vi "pco.camera_Simple_Example_IMAQ.vi"() -> ()   [LabVIEW 2019]
uses:
  pco.camera/Camera.lvclass
panel:
  out "rawImage":u16[][](array[numeric])
  out "Image":T1(plugin-control)
  in  "data_format":T2(ring)=enum."Mono16"
  in  "Image Index":u32 max=99
  out "Recorded Images":u32
  in  "Quit":bool
  in  "roiY1":u64=2 min=2 max=1040 step=1
  in  "roiX1":u64=2 min=2 max=1392 step=1
  in  "roiY0":u64=1 min=1 max=1039 step=1
  in  "roiX0":u64=1 min=1 max=1391 step=1
  out "Image Height":u16
  out "Image Width":u16
  in  "dwImgCount":u32=10 caption="Required Number of Images" max=4023
  out "Error":errorcluster {"code" format="%x"}
  # "This example shows a simple recording of an image sequence and the image access afterwards.\nIt is a good starting point for writing own applications.\nBut it will not be fail save, i.e. doesnt react on errors, just handles them forward to the end\n\nUsage:\nSelect your required image count before you start the program.\nOnce started, the camera class will be initialized and images will be recorded automatically.\nWhen acquisition has finished you can address the images and set a certain roi \nTo finish the program click on quit application, this will force fan exit of the camera class"
  # "pco.labview"
  # "Camera Setup"
  # "Recording Control"
  # "Parameters for image readout"
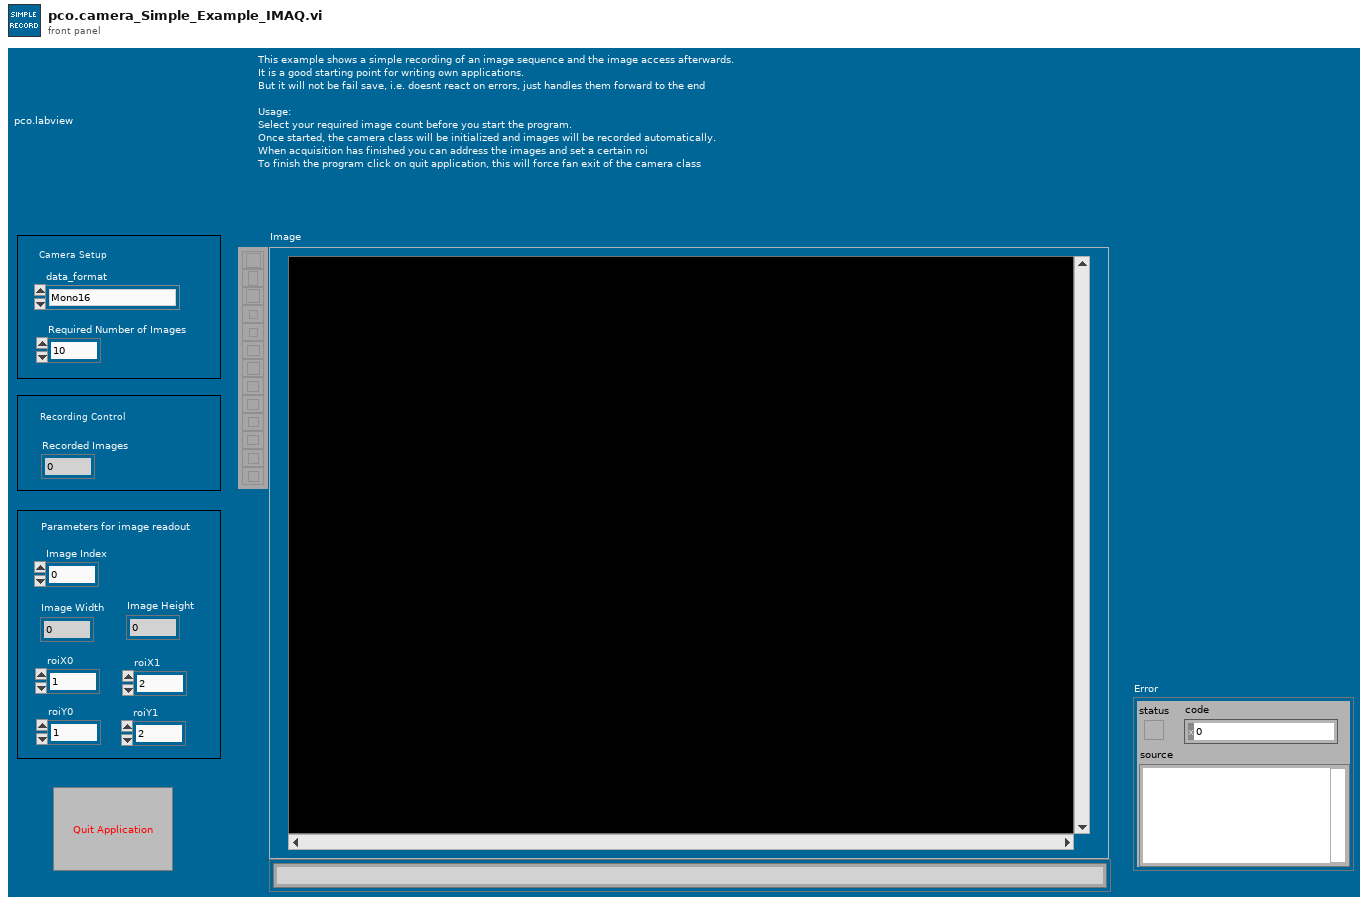
[diagram p1: front panel]
types:
  T1 = typedef "IMAQ Image.ctl" = refnum<image>
  T2 = enum16{"Undefined", "Mono8", "Mono16", "BGRA8", "RGBA8", "BGRA16", "RGBA16", "CompressedMono8"}
  T3 = enum8{"Enabled", "Disabled", "Disabled and Grayed Out"}
  T4 = enum16{"sequence", "sequence non blocking", "ring buffer", "fifo", "sequence_dpcore", "sequence_non_blocking_dpcore", "ring_buffer_dpcore", "fifo_dpcore", "tif", "multitif", "pcoraw", "b16", "dicom", "multidicom"}
  T5 = typedef "Image Type" = u32
  T6 = typedef "Camera.lvclass/binning.ctl" = cluster{"vert":u16, "horz":u16}
  T7 = cluster{"exposure_time_s":dbl, "delay_time_s":dbl, "roi":cluster{"x0":u64, "y0":u64, "x1":u64, "y1":u64}, "timestamp_mode":u16, "pixelrate":u32, "trigger_mode":u16, "acquire_mode":u16, "metadata_mode":u16, "noisefilter_mode":u16, "binning":T6}
  T8 = typedef "Color (U64)" = cluster{"Plane 3 (Blue)":u16, "Plane 2 (Green)":u16, "Plane 1 (Red)":u16, "Plane 4 (alpha)":u16}
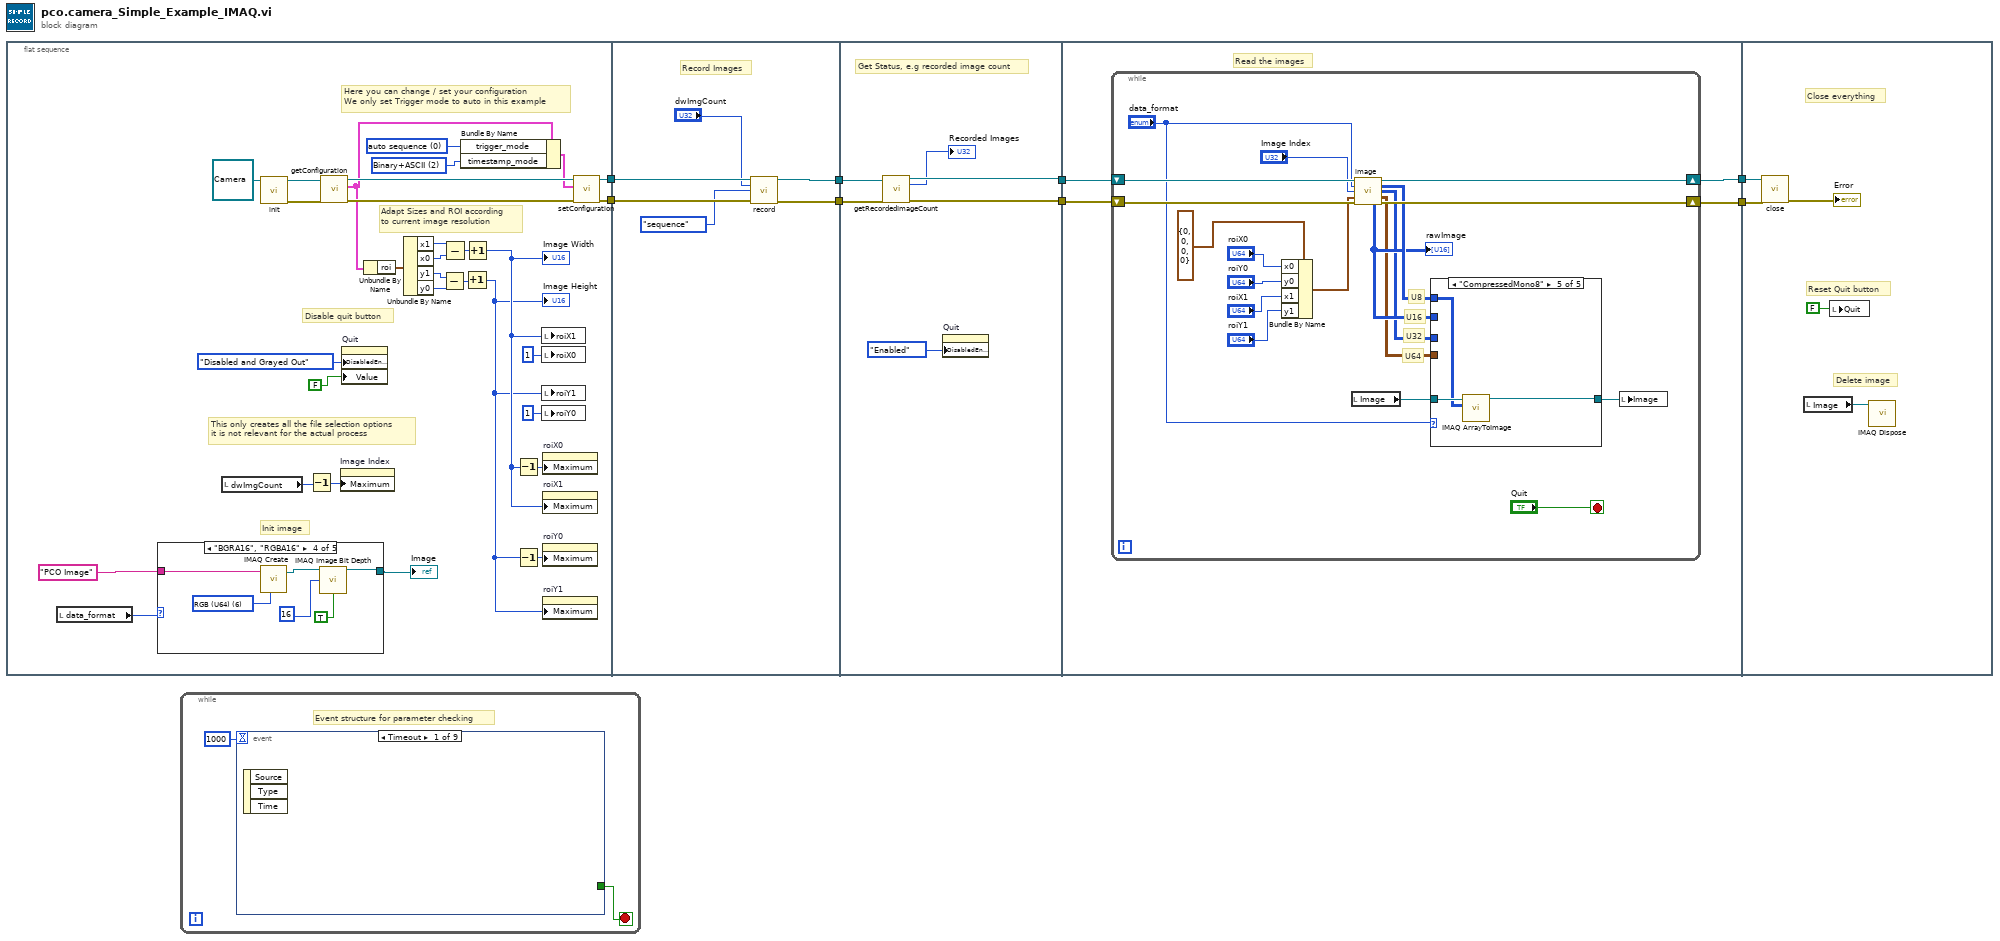
[diagram p0: block diagram]
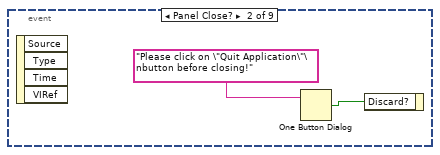
[diagram p2: hidden frame]
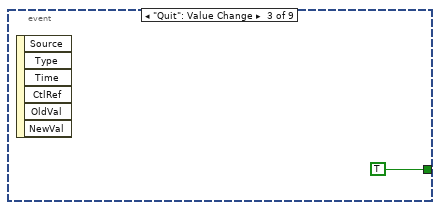
[diagram p3: hidden frame]
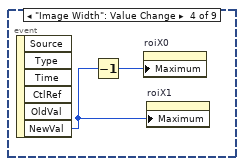
[diagram p4: hidden frame]
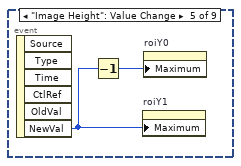
[diagram p5: hidden frame]
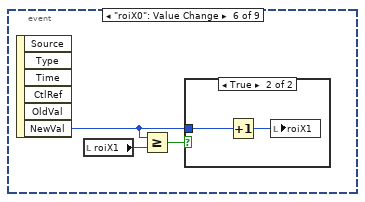
[diagram p6: hidden frame]
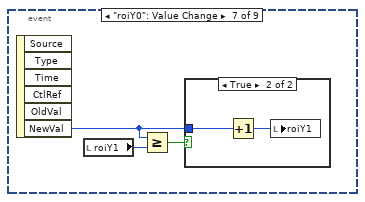
[diagram p8: hidden frame]
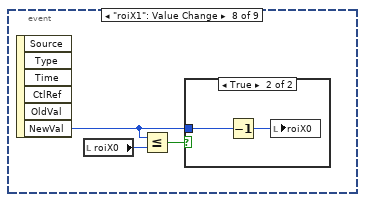
[diagram p10: hidden frame]
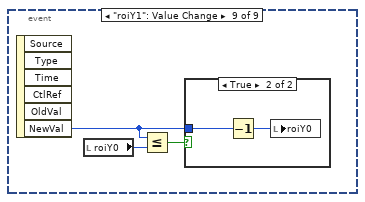
[diagram p12: hidden frame]
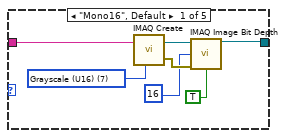
[diagram p14: hidden frame]
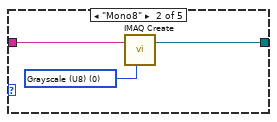
[diagram p15: hidden frame]
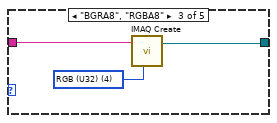
[diagram p16: hidden frame]
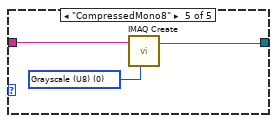
[diagram p17: hidden frame]
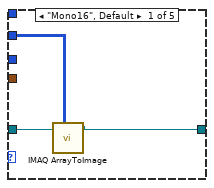
[diagram p18: hidden frame]
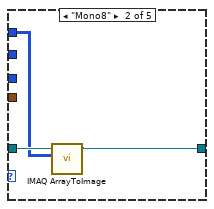
[diagram p19: hidden frame]
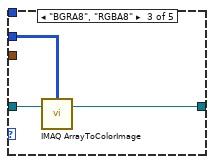
[diagram p20: hidden frame]
diagram:
  n1 = flat-sequence {
    tunnel: [w32] -> w8
    tunnel: [w31] -> w7
    tunnel: w8 -> [w67]
    tunnel: w7 -> [w66]
    tunnel: [w64] -> w6
    tunnel: [w63] -> w5
    tunnel: w6 -> [w73]
    tunnel: w5 -> [w72]
    tunnel: [w71] -> w4
    tunnel: [w70] -> w3
    tunnel: w4 -> [w76]
    tunnel: w3 -> [w77]
    tunnel: [w75] -> w2
    tunnel: [w74] -> w1
    tunnel: w2 -> [w114]
    tunnel: w1 -> [w113]
    frame #0 {
      w16 = u16 2 items=["OFF", "Binary", "Binary+ASCII", "ASCII"] ("TimestampMode")
      w36 = u16 0 items=["auto sequence"=0, "software trigger"=1, "external exposure start & software trigger"=2, "external exposure control"=3, "external synchronized"=4, "fast external exposure control"=5, "external CDS control"=6, "slow external exposure control"=7, "external synchronized HDSDI"=258] ("TriggerMode")
      # "Init image"
      # "This only creates all the file selection options\nit is not relevant for the actual process"
      # "Adapt Sizes and ROI according\nto current image resolution"
      # "Disable quit button"
      # "Here you can change / set your configuration\nWe only set Trigger mode to auto in this example"
      n2 = local read "data_format"() -> (w11:T2)
      n3 = case shown="\"BGRA16\", \"RGBA16\"" w11 {
        tunnel: "PCO Image" ("Image Name") -> [w45 w49 w51 w57 w60]
        tunnel: [w41 w47 w50 w53 w59] -> w10
        frame "Mono16", Default {
          w46 = T5 7 items=["Grayscale (U8)", "Grayscale (I16)", "Grayscale (SGL)", "Complex (CSG)", "RGB (U32)", "HSL (U32)", "RGB (U64)", "Grayscale (U16)"] ("Image Type")
          n4 = call "IMAQ Create"("Image Name"=w45, "Image Type"=w46) -> ("New Image"=w43:T1, "error out"=w42:errorcluster)  [unwired: 3 in]
          n5 = call "IMAQ Image Bit Depth"("Image"=w43, "Bit Depth (0)"=u32 16, "error in (no error)"=w42, "Get/Set Bit Depth? (Set)"=TRUE) -> ("Image Out"=w41:T1)  [unwired: 9 in, 2 out]
        }
        frame "Mono8" {
          w48 = T5 0 items=["Grayscale (U8)", "Grayscale (I16)", "Grayscale (SGL)", "Complex (CSG)", "RGB (U32)", "HSL (U32)", "RGB (U64)", "Grayscale (U16)"] ("Image Type")
          n6 = call "IMAQ Create"("Image Name"=w49, "Image Type"=w48) -> ("New Image"=w47:T1)  [unwired: 3 in, 1 out]
        }
        frame "BGRA8", "RGBA8" {
          w52 = T5 4 items=["Grayscale (U8)", "Grayscale (I16)", "Grayscale (SGL)", "Complex (CSG)", "RGB (U32)", "HSL (U32)", "RGB (U64)", "Grayscale (U16)"] ("Image Type")
          n7 = call "IMAQ Create"("Image Name"=w51, "Image Type"=w52) -> ("New Image"=w50:T1)  [unwired: 3 in, 1 out]
        }
        frame "BGRA16", "RGBA16" {
          w58 = T5 6 items=["Grayscale (U8)", "Grayscale (I16)", "Grayscale (SGL)", "Complex (CSG)", "RGB (U32)", "HSL (U32)", "RGB (U64)", "Grayscale (U16)"] ("Image Type")
          n8 = call "IMAQ Create"("Image Name"=w57, "Image Type"=w58) -> ("New Image"=w54:T1)  [unwired: 3 in, 1 out]
          n9 = call "IMAQ Image Bit Depth"("Image"=w54, "Bit Depth (0)"=u32 16, "Get/Set Bit Depth? (Set)"=TRUE) -> ("Image Out"=w53:T1)  [unwired: 10 in, 2 out]
        }
        frame "CompressedMono8" {
          w61 = T5 0 items=["Grayscale (U8)", "Grayscale (I16)", "Grayscale (SGL)", "Complex (CSG)", "RGB (U32)", "HSL (U32)", "RGB (U64)", "Grayscale (U16)"] ("Image Type")
          n10 = call "IMAQ Create"("Image Name"=w60, "Image Type"=w61) -> ("New Image"=w59:T1)  [unwired: 3 in, 1 out]
        }
      }
      "Image" <- w10
      n11 = local read "dwImgCount"() -> (w12:u32)
      n12 = call-dynamic "init.vi"("Camera in"=refnum<class "Camera.lvclass"> refnum ("PCOCamera in")) -> ("Camera out"=w38:refnum<class "Camera.lvclass">, "error out"=w37:errorcluster)  [unwired: 8 in]
      n13 = Decrement(x=w12) -> (x-1=w13:u32)
      n14 = call-dynamic "getConfiguration.vi"("error in (no error)"=w37, "Camera in"=w38) -> ("error out"=w34:errorcluster, "configuration"=w26:T7, "Camera out"=w35:refnum<class "Camera.lvclass">)  [unwired: 7 in]
      n15 = property on="Image Index" class="DigNum (strict)"("Maximum"=w13) -> ()  [unwired: 2 in, 2 out]
      n16 = property on="Quit" class="Bool (strict)"("DisabledEnum"=T3."Disabled and Grayed Out" ("Disabled"), "Value"=FALSE ("Stop")) -> ()  [unwired: 2 in, 2 out]
      n17 = Unbundle By Name(w26) -> ("roi"=w25:cluster{"x0":u64, "y0":u64, "x1":u64, "y1":u64})
      n18 = Unbundle By Name(w25) -> ("x1"=w23:u64, "x0"=w24:u64, "y1"=w21:u64, "y0"=w22:u64)
      n19 = Subtract(x=w21, y=w22) -> (x-y=w19:u64)
      n20 = Subtract(x=w23, y=w24) -> (x-y=w20:u64)
      n21 = Bundle By Name(cluster=w26, "trigger_mode"=w36, "timestamp_mode"=w16) -> (w33:T7)
      n22 = Increment(x=w19) -> (x+1=w17:u64)
      "Image Height" <- w17
      n23 = Increment(x=w20) -> (x+1=w18:u64)
      "Image Width" <- w18
      n24 = Decrement(x=w18) -> (x-1=w28:u64)
      n25 = Decrement(x=w17) -> (x-1=w27:u64)
      n26 = local write "roiX1"(w18) -> ()
      n27 = local write "roiX0"(u16 1 ("roiY0")) -> ()
      n28 = local write "roiY1"(w17) -> ()
      n29 = local write "roiY0"(u16 1 ("roiY0")) -> ()
      n30 = property on="roiX0" class="DigNum (strict)"("Maximum"=w28) -> ()  [unwired: 2 in, 2 out]
      n31 = property on="roiX1" class="DigNum (strict)"("Maximum"=w18) -> ()  [unwired: 2 in, 2 out]
      n32 = property on="roiY0" class="DigNum (strict)"("Maximum"=w27) -> ()  [unwired: 2 in, 2 out]
      n33 = property on="roiY1" class="DigNum (strict)"("Maximum"=w17) -> ()  [unwired: 2 in, 2 out]
      n34 = call-dynamic "setConfiguration.vi"("error in (no error)"=w34, "configuration"=w33, "Camera in"=w35) -> ("error out"=w31:errorcluster, "Camera out"=w32:refnum<class "Camera.lvclass">)  [unwired: 7 in]
    }
    frame #1 {
      # "Record Images"
      n35 = call-dynamic "record.vi"("Camera in"=w67, "num_images"="dwImgCount", "record_mode"=T4."sequence", "error in (no error)"=w66) -> ("Camera out"=w64:refnum<class "Camera.lvclass">, "error out"=w63:errorcluster)  [unwired: 10 in]
    }
    frame #2 {
      # "Get Status, e.g recorded image count"
      n36 = call-dynamic "getRecordedImageCount.vi"("Camera in"=w73, "error in (no error)"=w72) -> ("Camera out"=w71:refnum<class "Camera.lvclass">, "recorded_image_count"=→"Recorded Images":u32, "error out"=w70:errorcluster)  [unwired: 11 in]
      n37 = property on="Quit" class="Bool (strict)"("DisabledEnum"=T3."Enabled" ("Disabled")) -> ()  [unwired: 2 in, 2 out]
    }
    frame #3 {
      # "Read the images"
      n38 = while {
        shift-right: [w94] -> w75
        shift-left: w76 -> [w96]
        shift-right: [w89] -> w74
        shift-left: w77 -> [w95]
        stop <- "Quit" stop-if-true
        # "U64"
        # "U32"
        # "U16"
        # "U8"
        n39 = Bundle By Name(cluster=cluster{"x0":u64, "y0":u64, "x1":u64, "y1":u64} {"x0"=0, "y0"=0, "x1"=0, "y1"=0} ("roi"), "x0"="roiX0", "y0"="roiY0", "x1"="roiX1", "y1"="roiY1") -> (w88:cluster{"x0":u64, "y0":u64, "x1":u64, "y1":u64})
        n40 = local read "Image"() -> (w81:T1)
        n41 = call-dynamic "image.vi"("Camera in"=w96, "data_format"="data_format", "image_index"="Image Index", "roi"=w88, "error in (no error)"=w95) -> ("Camera out"=w94:refnum<class "Camera.lvclass">, "image (U8)"=w85:u8[][], "image (U32)"=w83:u32[][], "image (U64)"=w82:T8[][], "raw_image (U16)"=w84:u16[][], "error out"=w89:errorcluster)  [unwired: 3 in, 2 out]
        "rawImage" <- w84
        n42 = case shown="\"CompressedMono8\"" "data_format" {
          tunnel: w81 -> [w99 w102 w105 w108 w111]
          tunnel: [w97 w100 w104 w106 w110] -> w80
          tunnel: w82 -> [_ _ _ w107 _]
          tunnel: w83 -> [_ _ w103 _ _]
          tunnel: w85 -> [_ w101 _ _ w109]
          tunnel: w84 -> [w98 _ _ _ _]
          frame "Mono16", Default {
            n43 = call "IMAQ ArrayToImage"("Image Pixels (U16)"=w98, "Image"=w99) -> ("Image Out"=w97:T1)  [unwired: 8 in, 1 out]
          }
          frame "Mono8" {
            n44 = call "IMAQ ArrayToImage"("Image Pixels (U8)"=w101, "Image"=w102) -> ("Image Out"=w100:T1)  [unwired: 8 in, 1 out]
          }
          frame "BGRA8", "RGBA8" {
            n45 = call "IMAQ ArrayToColorImage"("Image Pixels (U32)"=w103, "Image"=w105) -> ("Image Out"=w104:T1)  [unwired: 3 in, 1 out]
          }
          frame "BGRA16", "RGBA16" {
            n46 = call "IMAQ ArrayToColorImage"("Image"=w108, "Image Pixels (U64)"=w107) -> ("Image Out"=w106:T1)  [unwired: 3 in, 1 out]
          }
          frame "CompressedMono8" {
            n47 = call "IMAQ ArrayToImage"("Image Pixels (U8)"=w109, "Image"=w111) -> ("Image Out"=w110:T1)  [unwired: 8 in, 1 out]
          }
        }
        n48 = local write "Image"(w80) -> ()
      }
    }
    frame #4 {
      # "Delete image"
      # "Reset Quit button"
      # "Close everything"
      n49 = call-dynamic "close.vi"("error in (no error)"=w113, "Camera in"=w114) -> ("error out"=→"Error":errorcluster)  [unwired: 9 in]
      n50 = local read "Image"() -> (w112:T1)
      n51 = local write "Quit"(FALSE ("Stop")) -> ()
      n52 = call "IMAQ Dispose"("Image"=w112) -> ()  [unwired: 5 in, 1 out]
    }
  }
  n53 = while {
    stop <- w117 stop-if-true
    # "Event structure for parameter checking"
    n54 = event shown="[0] Timeout" {
      selector: _ -> [_ _ _ _ _ _ _ _ _]
      dyn-events: _ -> [_ _ _ _ _ _ _ _ _]
      timeout: 1000 -> [_ _ _ _ _ _ _ _ _]
      tunnel: [_ _ TRUE _ _ _ _ _ _] -> w117
      event Timeout {
        n55 = event-data() -> ()  [unwired: 1 in, 3 out]
      }
      event Panel Close? {
        n56 = event-data() -> ()  [unwired: 1 in, 4 out]
        n57 = One Button Dialog(message="Please click on \"Quit Application\"\nbutton before closing!") -> (true=w119:bool)  [unwired: 1 in]
        n58 = event-data("Discard?"=w119) -> ()  [unwired: 1 in, 1 out]
      }
      event "Quit": Value Change {
        n59 = event-data() -> ()  [unwired: 1 in, 6 out]
      }
      event "Image Width": Value Change {
        n60 = event-data() -> ("NewVal"=w122:u16)  [unwired: 1 in, 5 out]
        n61 = Decrement(x=w122) -> (x-1=w123:u16)
        n62 = property on="roiX0" class="DigNum (strict)"("Maximum"=w123) -> ()  [unwired: 2 in, 2 out]
        n63 = property on="roiX1" class="DigNum (strict)"("Maximum"=w122) -> ()  [unwired: 2 in, 2 out]
      }
      event "Image Height": Value Change {
        n64 = event-data() -> ("NewVal"=w124:u16)  [unwired: 1 in, 5 out]
        n65 = Decrement(x=w124) -> (x-1=w125:u16)
        n66 = property on="roiY1" class="DigNum (strict)"("Maximum"=w124) -> ()  [unwired: 2 in, 2 out]
        n67 = property on="roiY0" class="DigNum (strict)"("Maximum"=w125) -> ()  [unwired: 2 in, 2 out]
      }
      event "roiX0": Value Change {
        n68 = event-data() -> ("NewVal"=w126:u64)  [unwired: 1 in, 5 out]
        n69 = local read "roiX1"() -> (w128:u64)
        n70 = Greater Or Equal?(x=w126, y=w128) -> (x >= y?=w127:bool)
        n71 = case shown="True" w127 {
          tunnel: w126 -> [_ w130]
          frame False {
          }
          frame True {
            n72 = Increment(x=w130) -> (x+1=w129:u64)
            n73 = local write "roiX1"(w129) -> ()
          }
        }
      }
      event "roiY0": Value Change {
        n74 = event-data() -> ("NewVal"=w131:u64)  [unwired: 1 in, 5 out]
        n75 = local read "roiY1"() -> (w133:u64)
        n76 = Greater Or Equal?(x=w131, y=w133) -> (x >= y?=w132:bool)
        n77 = case shown="True" w132 {
          tunnel: w131 -> [_ w135]
          frame False {
          }
          frame True {
            n78 = Increment(x=w135) -> (x+1=w134:u64)
            n79 = local write "roiY1"(w134) -> ()
          }
        }
      }
      event "roiX1": Value Change {
        n80 = event-data() -> ("NewVal"=w136:u64)  [unwired: 1 in, 5 out]
        n81 = local read "roiX0"() -> (w138:u64)
        n82 = Less Or Equal?(x=w136, y=w138) -> (x <= y?=w137:bool)
        n83 = case shown="True" w137 {
          tunnel: w136 -> [_ w140]
          frame False {
          }
          frame True {
            n84 = Decrement(x=w140) -> (x-1=w139:u64)
            n85 = local write "roiX0"(w139) -> ()
          }
        }
      }
      event "roiY1": Value Change {
        n86 = event-data() -> ("NewVal"=w141:u64)  [unwired: 1 in, 5 out]
        n87 = local read "roiY0"() -> (w143:u64)
        n88 = Less Or Equal?(x=w141, y=w143) -> (x <= y?=w142:bool)
        n89 = case shown="True" w142 {
          tunnel: w141 -> [_ w145]
          frame False {
          }
          frame True {
            n90 = Decrement(x=w145) -> (x-1=w144:u64)
            n91 = local write "roiY0"(w144) -> ()
          }
        }
      }
    }
  }
